vi "Convert April Tag Data types.vi"(10 "Detections in":T2[](array[typedef])) -> (3 "tags":T1(array[cluster]))   [LabVIEW 2025]
uses:
  <vilib>/serenial/G Augmented-Reality Toolkit/g_ar_toolkit.feature_detection/Apriltag Detector/Detection.ctl
  <vilib>/serenial/G Augmented-Reality Toolkit/g_ar_toolkit.common/Image Point (Float).ctl
  <vilib>/serenial/G Augmented-Reality Toolkit/g_ar_toolkit.common/Quad Corners.ctl
  <vilib>/serenial/G Augmented-Reality Toolkit/g_ar_toolkit.common/g_ar_toolkit.common.lvlib
  <vilib>/serenial/G Augmented-Reality Toolkit/g_ar_toolkit.feature_detection/Apriltag Detector/AprilTag Detector.lvclass
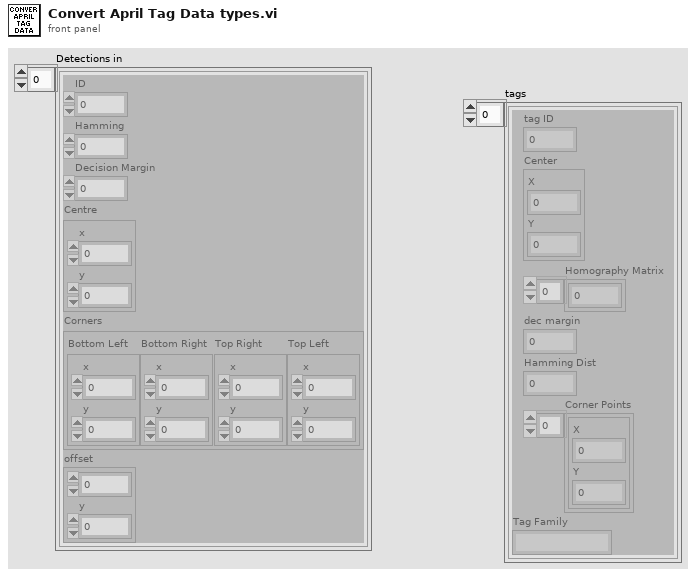
[diagram p1: front panel]
types:
  T1 = cluster{"tag ID":i32, "Center":cluster{"X":dbl, "Y":dbl}, "Homography Matrix":dbl[], "dec margin":dbl, "Hamming Dist":i32, "Corner Points":cluster{"X":dbl, "Y":dbl}[], "Tag Family":string}[]
  T2 = typedef "g_ar_toolkit.feature_detection.lvlib/AprilTag Detector.lvclass/Detection.ctl" = cluster{"ID":i32, "Hamming":i32, "Decision Margin":sgl, "Centre":T3, "Corners":T4, "offset":cluster{dbl, "y":dbl}}
  T3 = typedef "g_ar_toolkit.common.lvlib/Image Point (Float).ctl" = cluster{"x":dbl, "y":dbl}
  T4 = typedef "g_ar_toolkit.common.lvlib/Quad Corners.ctl" = cluster{"Bottom Left":T3, "Bottom Right":T3, "Top Right":T3, "Top Left":T3}
  T5 = cluster{"ID":i32, "Centre":T3, dbl[], "Decision Margin":sgl, "Hamming":i32, "Corners":T3[], string}
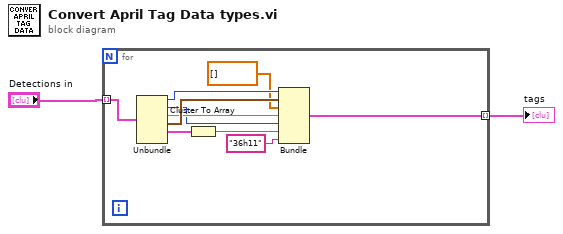
[diagram p0: block diagram]
diagram:
  n1 = for {
    tunnel: "Detections in" -> [w12] mode=indexing
    tunnel: [w9] -> w1 mode=indexing
    n2 = Unbundle(w12) -> ("ID"=w11:i32, "Hamming"=w7:i32, "Decision Margin"=w8:sgl, "Centre"=w10:T3, "Corners"=w5:T4)  [unwired: 1 out]
    n3 = Cluster To Array(cluster=w5) -> (array=w4:T3[])
    n4 = Bundle("ID"=w11, "Centre"=w10, dbl[] [], "Decision Margin"=w8, "Hamming"=w7, "Corners"=w4, "36h11") -> (w9:T5)  [unwired: 1 in]
  }
  "tags" <- w1
